vi "Fill FN - Hydration Spray (SubVI).vi"(0 "Signals IN":T2={"Dispense"=FALSE, "Fill"=FALSE, "Spray"=FALSE, "Drain"=TRUE, "Complete"=FALSE, "Fill Error"=FALSE, "Dispense Error"=FALSE, "Fill Timeout"=FALSE, "Dispense Timeout"=FALSE}, 1 "Values IN":T1 {"Drain Time (s)" format="%.2f"; "Drain Rate (g/sec)" format="%.2f"}, 3 "Settings":T3={"ON Settings"={"Enable Dynamic Setpoint?"=TRUE, "Enable Dynamic Dispense Time?"=TRUE, "Enable Drain Rate Functions"=TRUE, "Dispense Sample Time (s)"=0.5, "Dispense Slope Ave"=0, "ON Timeout (sec)"=600.0, "1st Setpoint (% of Target)"=0.0, "2nd Setpoint (% of Target)"=0.0, "3rd Setpoint (% of Target)"=0.0, "Measure Dispense Delay (sec)"=0.0, "Settle Slope Sample Time (s)"=0.0}, "OFF Settings"={"Drain Sample Time (s)"=0.5, "Drain Rate Ave Size"=5, "Drain Rate Limits (± g/sec)"=10.0, "Level Slope Range (± g/sec)"=0.25, "OFF Timeout (sec)"=0.0, "Near SP Slope Level (± g/sec)"=0.01, "Near Setpoint Threshold (%)"=95.0}, "Overshoot Settings"={"Time Limit (s)"=60.0, "Container MAX (g)"=1500.0, "Max FILL Slope (+/- g/sec)"=10.0, "% Overshot to Enable (>)"=0.25}, "FILL Timeout (s)"=300.0, "Full Settle Time (s)"=20.0, "Pre-Hydrate \nSpray Time (s)"=10.0, "Pre-Hydrate \nWait Time (s)"=30.0}, 5 "Fill Case Change?":bool) -> (14 "Signals OUT":T2, 15 "Values OUT":T1, 19 "Case Complete":bool)   [LabVIEW 2012]
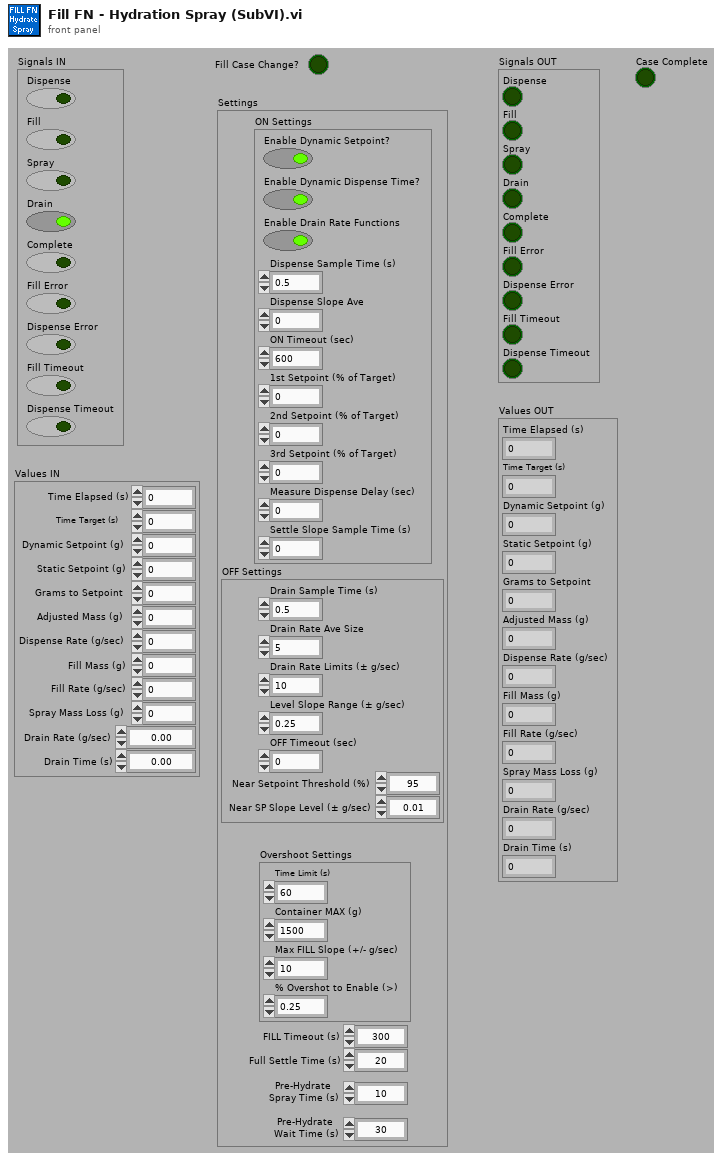
[diagram p1: front panel]
types:
  T1 = cluster{"Time Elapsed (s)":dbl, "Time Target (s)":dbl, "Dynamic Setpoint (g)":dbl, "Static Setpoint (g)":dbl, "Grams to Setpoint":dbl, "Adjusted Mass (g)":dbl, "Dispense Rate (g/sec)":dbl, "Fill Mass (g)":dbl, "Fill Rate (g/sec)":dbl, "Spray Mass Loss (g)":dbl, "Drain Rate (g/sec)":dbl, "Drain Time (s)":dbl}
  T2 = cluster{"Dispense":bool, "Fill":bool, "Spray":bool, "Drain":bool, "Complete":bool, "Fill Error":bool, "Dispense Error":bool, "Fill Timeout":bool, "Dispense Timeout":bool}
  T3 = cluster{"ON Settings":cluster{"Enable Dynamic Setpoint?":bool, "Enable Dynamic Dispense Time?":bool, "Enable Drain Rate Functions":bool, "Dispense Sample Time (s)":dbl, "Dispense Slope Ave":i32, "ON Timeout (sec)":dbl, "1st Setpoint (% of Target)":dbl, "2nd Setpoint (% of Target)":dbl, "3rd Setpoint (% of Target)":dbl, "Measure Dispense Delay (sec)":dbl, "Settle Slope Sample Time (s)":dbl}, "OFF Settings":cluster{"Drain Sample Time (s)":dbl, "Drain Rate Ave Size":i32, "Drain Rate Limits (± g/sec)":dbl, "Level Slope Range (± g/sec)":dbl, "OFF Timeout (sec)":dbl, "Near SP Slope Level (± g/sec)":dbl, "Near Setpoint Threshold (%)":dbl}, "Overshoot Settings":cluster{"Time Limit (s)":dbl, "Container MAX (g)":dbl, "Max FILL Slope (+/- g/sec)":dbl, "% Overshot to Enable (>)":dbl}, "FILL Timeout (s)":dbl, "Full Settle Time (s)":dbl, "Pre-Hydrate \nSpray Time (s)":dbl, "Pre-Hydrate \nWait Time (s)":dbl}
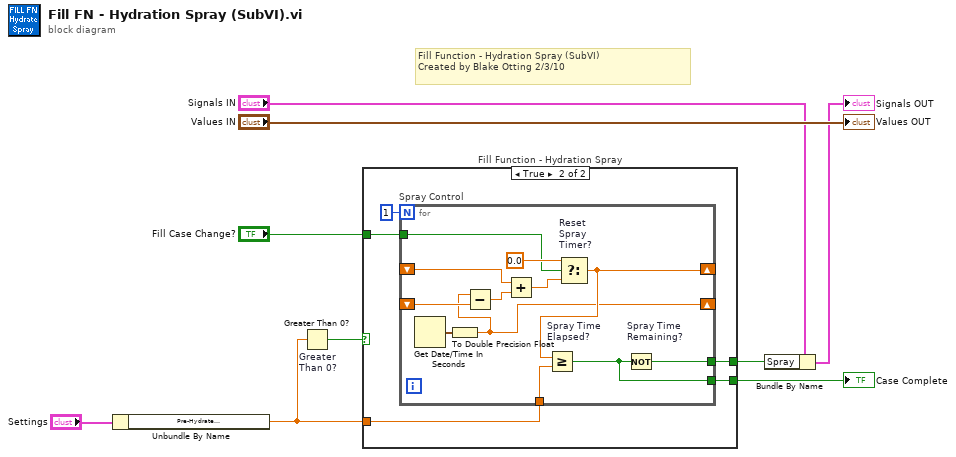
[diagram p0: block diagram]
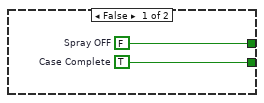
[diagram p2: hidden frame]
diagram:
  # "Fill Function - Hydration Spray (SubVI)\nCreated by Blake Otting 2/3/10"
  n1 = Unbundle By Name("Settings") -> ("Pre-Hydrate \nSpray Time (s)"=w2:dbl)
  n2 = Greater Than 0? "Greater\nThan 0?"(x=w2) -> (x > 0?=w4:bool)
  n3 = case "Fill Function - Hydration Spray" shown="True" w4 {
    tunnel: "Fill Case Change?" -> [_ w15]
    tunnel: w2 -> [_ w14]
    tunnel: [w11 w13] -> w8
    tunnel: [w10 w12] -> w9
    frame False {
      w11 = TRUE  # Case Complete
      w10 = FALSE  # Spray OFF
    }
    frame True {
      n4 = for "Spray Control" {
        N: 1 -> [_]
        shift-right: [w21] -> _
        shift-left: _ -> [w28]
        shift-right: [w20] -> _
        shift-left: _ -> [w25]
        tunnel: w15 -> [w19]
        tunnel: w14 -> [w22]
        tunnel: [w17] -> w13
        tunnel: [w18] -> w12
        n5 = Get Date/Time In Seconds() -> (seconds since 1Jan1904=w27:timestamp)
        n6 = To Double Precision Float(number=w27) -> (double precision float=w20:dbl)
        n7 = Subtract(x=w20, y=w25) -> (x-y=w24:dbl)
        n8 = Add(x=w28, y=w24) -> (x+y=w26:dbl)
        n9 = Select "Reset\nSpray\nTimer?"(t=0.0, s=w19, f=w26) -> (s? t:f=w21:dbl)
        n10 = Greater Or Equal? "Spray Time\nElapsed?"(x=w21, y=w22) -> (x >= y?=w17:bool)
        n11 = Not "Spray Time\nRemaining?"(x=w17) -> (.not. x?=w18:bool)
      }
    }
  }
  "Case Complete" <- w8
  n12 = Bundle By Name(cluster="Signals IN", "Spray"=w9) -> (→"Signals OUT":T2)
  "Values OUT" <- "Values IN"
